vi "Enum from Value.vi"(10 "Value":i32) -> (2 "Enumeration":T1)   [LabVIEW 2020, in "ConnectStatus.lvlib"]
uses:
  ConnectStatus.lvlib
  Enumeration.ctl
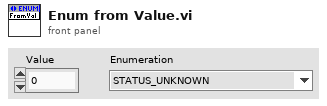
[diagram p1: front panel]
types:
  T1 = typedef "ConnectStatus.lvlib/Enumeration.ctl" = enum16{"STATUS_UNKNOWN", "STATUS_SUCCESS", "STATUS_ERROR", "STATUS_BAD_CONFIG", "STATUS_BAD_SYSTEM", "STATUS_BAD_CLUSTER", "STATUS_NOT_ALLOWED"}
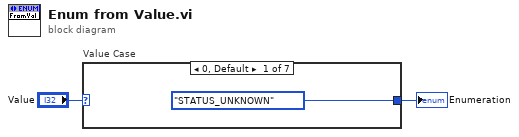
[diagram p0: block diagram]
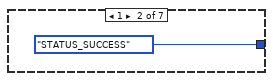
[diagram p2: hidden frame]
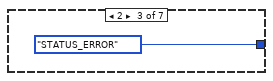
[diagram p3: hidden frame]
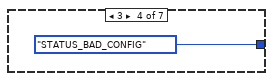
[diagram p4: hidden frame]
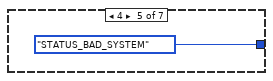
[diagram p5: hidden frame]
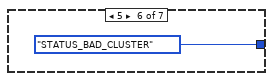
[diagram p6: hidden frame]
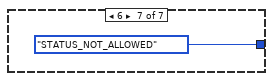
[diagram p7: hidden frame]
diagram:
  n1 = case "Value Case" shown="0, Default" "Value" {
    tunnel: [Enumeration."STATUS_UNKNOWN" ("Enumeration") Enumeration."STATUS_SUCCESS" ("Enumeration") Enumeration."STATUS_ERROR" ("Enumeration") Enumeration."STATUS_BAD_CONFIG" ("Enumeration") Enumeration."STATUS_BAD_SYSTEM" ("Enumeration") Enumeration."STATUS_BAD_CLUSTER" ("Enumeration") Enumeration."STATUS_NOT_ALLOWED" ("Enumeration")] -> w1
    frame 0, Default {
    }
    frame 1 {
    }
    frame 2 {
    }
    frame 3 {
    }
    frame 4 {
    }
    frame 5 {
    }
    frame 6 {
    }
  }
  "Enumeration" <- w1
